vi "sendTelFromTcpClientAndGetTelemetry.vi"(8 "error in (no error)":errorcluster, 10 "tel connection ID in":refnum<k5>, 11 "TcpServer in":refnum<class "TcpServer.lvclass">) -> (0 "error out":errorcluster, 1 "telemetry sent":string[](array[string]), 2 "tel connection ID out":refnum<k5>, 3 "TcpServer out":refnum<class "TcpServer.lvclass">, 4 "telemetry received":string[](array[string]))   [LabVIEW 2018]
doc: "Generate 10 elements of telemetry and send them to TCP server. Then, this telemetry is read."
uses:
  src/TcpServer/TcpServer.lvclass
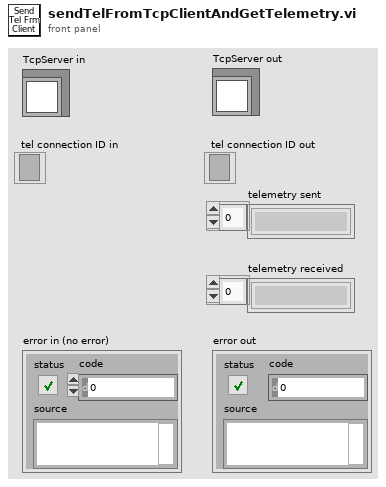
[diagram p1: front panel]
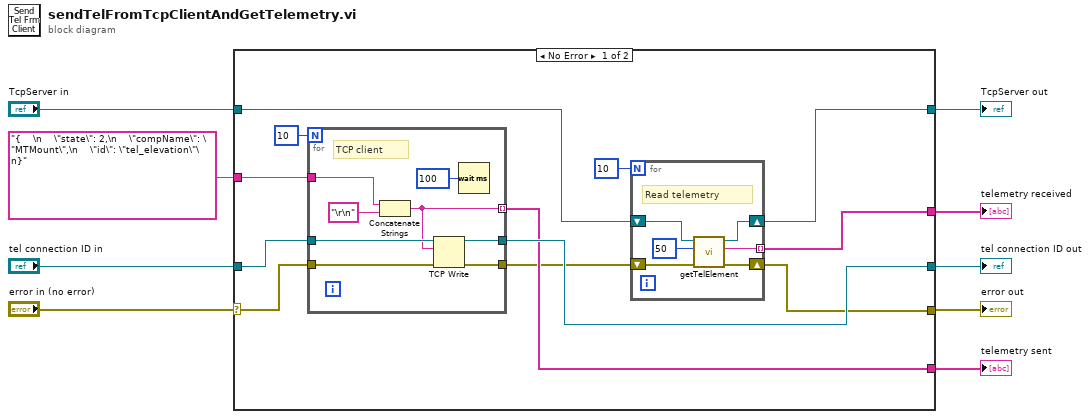
[diagram p0: block diagram]
diagram:
  n1 = case shown="No Error" "error in (no error)" {
    selector: "error in (no error)" -> [w18 w38]
    tunnel: [w21 w36] -> w9
    tunnel: [w20 w37] -> w8
    tunnel: "TcpServer in" -> [w19 w36]
    tunnel: [w17 _] -> w5
    tunnel: [w16 _] -> w1
    tunnel: [w14 w38] -> w4
    tunnel: "tel connection ID in" -> [w11 w37]
    tunnel: "{    \n    \"state\": 2,\n    \"compName\": \"MTMount\",\n    \"id\": \"tel_elevation\"\n}" ("Display") -> [w10 _]
    frame No Error {
      n2 = for {
        N: 10 -> [_]
        tunnel: [w31] -> w20
        tunnel: w11 -> [w33]
        tunnel: [w30] -> w12
        tunnel: w18 -> [w32]
        tunnel: w10 -> [w29]
        tunnel: [w28] -> w17 mode=indexing
        # "TCP client"
        n3 = Concatenate Strings(w29, "\r\n" ("string")) -> (w28:string)
        n4 = TCP Write(connection ID=w33, data in=w28, error in (no error)=w32) -> (connection ID out=w31:refnum<k5>, error out=w30:errorcluster)  [unwired: 1 in, 1 out]
        n5 = Wait (ms)(milliseconds to wait=u32 100) -> ()  [unwired: 1 out]
      }
      n6 = for {
        N: 10 -> [_]
        shift-right: [w26] -> w14
        shift-left: w12 -> [w27]
        shift-right: [w24] -> w21
        shift-left: w19 -> [w25]
        tunnel: [w23] -> w16 mode=indexing
        # "Read telemetry"
        n7 = call "getTelElement.vi"("error in (no error)"=w27, "timeoutQueueTcpClientFromDds"=50, "TcpServer in"=w25) -> ("error out"=w26:errorcluster, "tcpPacket"=w23:string, "TcpServer out"=w24:refnum<class "TcpServer.lvclass">)  [unwired: 5 in, 1 out]
      }
    }
    frame Error {
    }
  }
  "TcpServer out" <- w9
  "tel connection ID out" <- w8
  "telemetry sent" <- w5
  "error out" <- w4
  "telemetry received" <- w1
